vi "init.vi"(8 "error in (no error)":errorcluster, 11 "Thermocouple in":refnum<class "Thermocouple.lvclass">) -> (0 "error out":errorcluster, 3 "Thermocouple out":refnum<class "Thermocouple.lvclass">)   [LabVIEW 2013, in "Thermocouple.lvclass"]
uses:
  Thermocouple.lvclass
  Configuration/Thermocouple.ctl
  Configuration/MotorOverheatTemperature.ctl
  Thermocouple.lvclass/Thermocouple.ctl
  ConfigurationThisComponent/ConfigurationThisComponent.lvclass
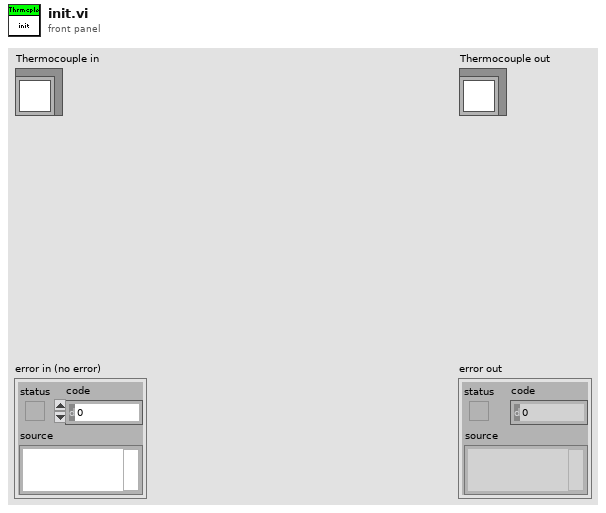
[diagram p1: front panel]
types:
  T1 = typedef "Thermocouple.ctl" = cluster{"Thermocouple Conversion":dbl[unit], "Motor Overheat Temperature":T2, "Ambient Temperature":T2}
  T2 = typedef "MotorOverheatTemperature.ctl" = dbl[unit]
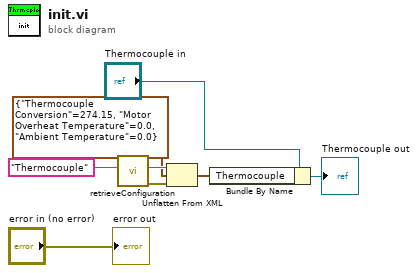
[diagram p0: block diagram]
diagram:
  n1 = call "retrieveConfiguration.vi"("configName"="Thermocouple") -> ("error out"=w5:errorcluster, "xmlConfig"=w6:string)  [unwired: 8 in, 1 out]
  n2 = Unflatten From XML(xml string=w6, type=T1 {"Thermocouple Conversion"=274.15, "Motor Overheat Temperature"=0.0, "Ambient Temperature"=0.0} ("Thermocouple"), error in (no error)=w5) -> (value=w3:T1)  [unwired: 1 out]
  n3 = Bundle By Name(cluster="Thermocouple in", "Thermocouple"=w3) -> (→"Thermocouple out":refnum<class "Thermocouple.lvclass">)
  "error out" <- "error in (no error)"
